vi "hasFrame.vi"(8 "Error In":errorcluster, 11 "QLineEdit In":refnum<class "QLineEdit.lvclass">) -> (0 "Error Out":errorcluster, 2 "Value":bool, 3 "QLineEdit Out":refnum<class "QLineEdit.lvclass">)   [LabVIEW 2014, in "QLineEdit.lvclass"]
doc: "LabVIEW-specific documentation is not yet available. See <b>https://doc.qt.io/qt-5/qlineedit.html#hasFrame</b>"
uses:
  QLineEdit.lvclass
  LQ Core/LQIdentity/LQIdentity.lvclass/LQIdentity.ctl
  LQ Core/LQ Core.lvlib
  LQ Core/LQIdentity/LQIdentity.lvclass
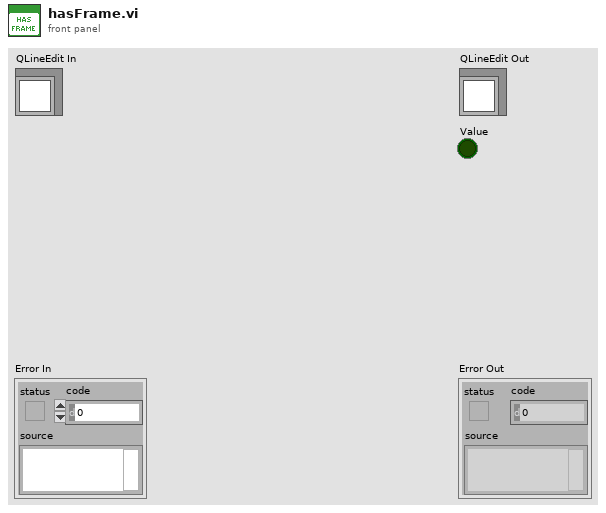
[diagram p1: front panel]
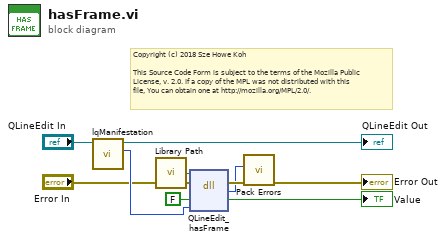
[diagram p0: block diagram]
diagram:
  # "Copyright (c) 2018 Sze Howe Koh\n\nThis Source Code Form is subject to the terms of the Mozilla Public\nLicense, v. 2.0. If a copy of the MPL was not distributed with this\nfile, You can obtain one at http://mozilla.org/MPL/2.0/."
  n1 = call "lqManifestation.vi"("LQIdentity in"="QLineEdit In") -> ("Manifestation"=w5:u64, "LQIdentity out"=→"QLineEdit Out":refnum<class "QLineEdit.lvclass">)  [unwired: 9 in]
  n2 = call "Library Path.vi"() -> ("Library Path"=w6:path)
  n3 = dll-call lib="?" fn="QLineEdit_hasFrame"(path in=w6, error in="Error In", "_retVal"=FALSE, "_instance"=w5) -> (error out=w3:errorcluster, w1:i32, "_retVal"=→"Value":bool)  [unwired: 2 in, 1 out]
  n4 = call "Pack Errors.vi"("Error In"=w3, "Error Code"=w1) -> ("Error Out"=→"Error Out":errorcluster)  [unwired: 9 in]
